vi "testTimestampParsingNoTimeZone.vi"(8 "error in (no error)":errorcluster, 11 "TestCase in":refnum<class "EasyXMLTest.lvclass">) -> (0 "error out":errorcluster, 3 "TestCase out":refnum<class "EasyXMLTest.lvclass">)   [LabVIEW 2013, in "EasyXMLTest.lvclass"]
doc: "Verify that error in is not overwritten"
uses:
  EasyXMLTest.lvclass
panel:
  out "dateTime out":timestamp
  out "Produced Data":variant
  out "Expected Data":variant
  out "XML String":string
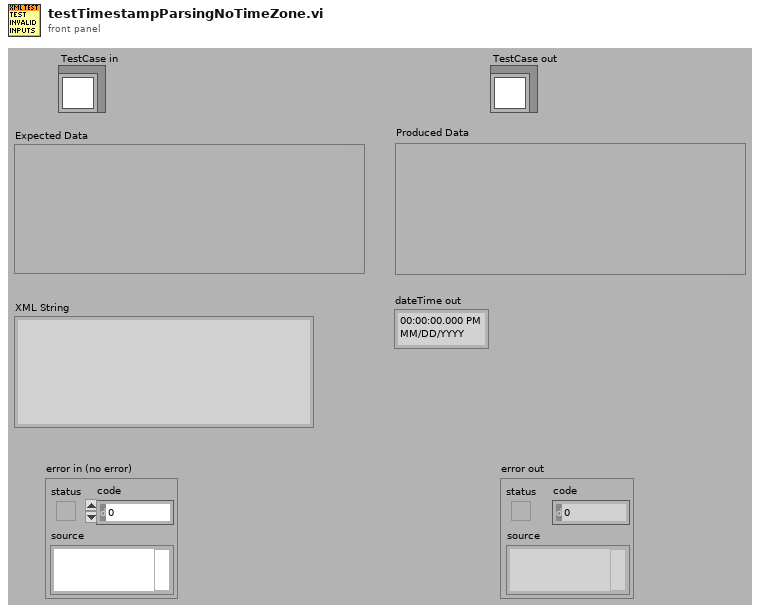
[diagram p1: front panel]
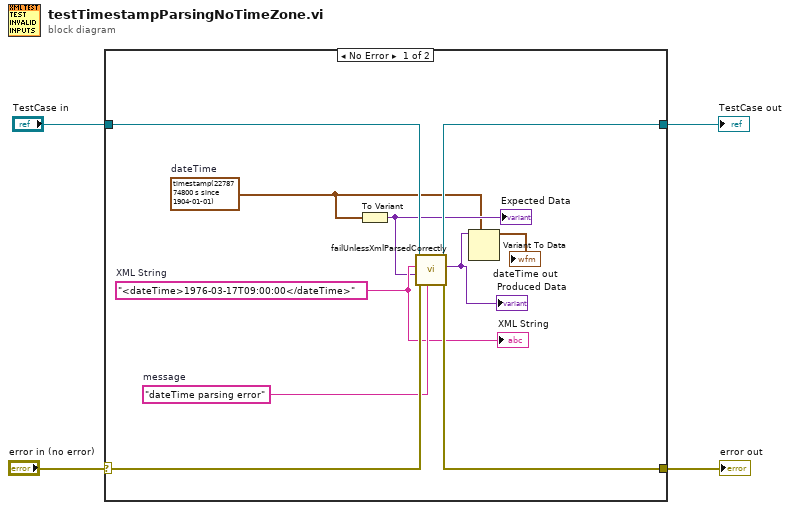
[diagram p0: block diagram]
diagram:
  n1 = case shown="No Error" "error in (no error)" {
    selector: "error in (no error)" -> [w13 w16]
    tunnel: [w12 w16] -> w2
    tunnel: [w11 w15] -> w1
    tunnel: "TestCase in" -> [w14 w15]
    frame No Error {
      w5 = timestamp(2278774800 s since 1904-01-01)  # dateTime
      w9 = "<dateTime>1976-03-17T09:00:00</dateTime>"  # XML String
      w10 = "dateTime parsing error"  # message
      n2 = To Variant(anything=w5) -> (Variant=w8:variant)
      "Expected Data" <- w8
      n3 = call "failUnlessXmlParsedCorrectly.vi"("message (\"\")"=w10, "error in"=w13, "Expected Data"=w8, "XML String"=w9, "reference in"=w14) -> ("error out"=w12:errorcluster, "Produced Data"=w7:variant, "reference in"=w11:refnum<class "EasyXMLTest.lvclass">)  [unwired: 4 in]
      "Produced Data" <- w7
      n4 = Variant To Data(type=w5, Variant=w7) -> (data=→"dateTime out":timestamp)  [unwired: 1 in, 1 out]
      "XML String" <- w9
    }
    frame Error {
    }
  }
  "error out" <- w2
  "TestCase out" <- w1
